vi "build map_object_key.vi"(10 "objectClassHandle":u64, 11 "instanceId":i32) -> (3 "object_map_key":T1)   [LabVIEW 2019, in "HLA Custom Device Engine.lvlib"]
uses:
  HLA Custom Device Engine.lvlib
  map_object_key.ctl
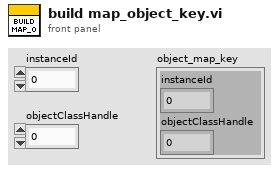
[diagram p1: front panel]
types:
  T1 = typedef "HLA Custom Device Engine.lvlib/map_object_key.ctl" = cluster{"instanceId":i32, "objectClassHandle":u64}
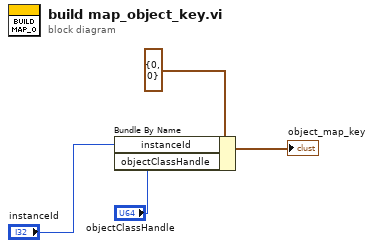
[diagram p0: block diagram]
diagram:
  n1 = Bundle By Name(cluster=T1 {"instanceId"=0, "objectClassHandle"=0} ("input cluster"), "instanceId"="instanceId", "objectClassHandle"="objectClassHandle") -> (→"object_map_key":T1)
